vi "TCP PXI DAQ Listener.vi"(0 "port":u16, 11 "error in (no error)":errorcluster) -> (4 "connection ID":refnum<k5>, 8 "Connected?":bool, 15 "error out":errorcluster)   [LabVIEW 2015]
uses:
  DAQ Engine VIs/PXI Globals.vi
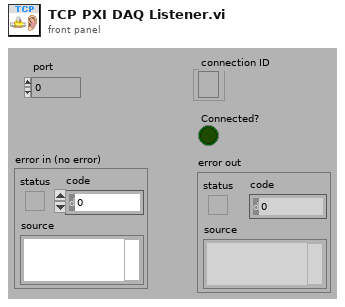
[diagram p1: front panel]
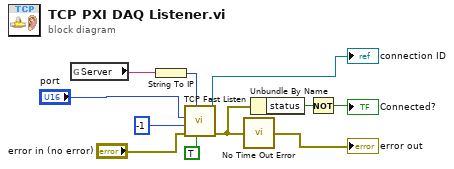
[diagram p0: block diagram]
diagram:
  n1 = global read "PXI Globals.vi" "Server"() -> (w4:string)
  n2 = String To IP(1:w4) -> (0:w6:u32)
  n3 = call "TCP Fast Listen.vi"("TCP_NODELAY (true)"=TRUE, "net address"=w6, "error in (no error)"="error in (no error)", "timeout ms (wait forever: -1)"=-1, "port"="port") -> ("error out"=w8:errorcluster, "connection ID"=→"connection ID":refnum<k5>)  [unwired: 3 in, 2 out]
  n4 = call "No Time Out Error.vi"("error in"=w8) -> ("error out"=→"error out":errorcluster)  [unwired: 14 in]
  n5 = Unbundle By Name(w8) -> ("status"=w9:bool)
  n6 = Not(x=w9) -> (.not. x?=→"Connected?":bool)
